vi "ReversedEngineering GetObjectRefsFromPanel.vi"(1 "Path":path, 5 "error in (no error)":errorcluster) -> (15 "objectRefsFound":path[](array[path]), 16 "array":bool[](array[boolean]), 19 "error out":errorcluster)   [LabVIEW 2014]
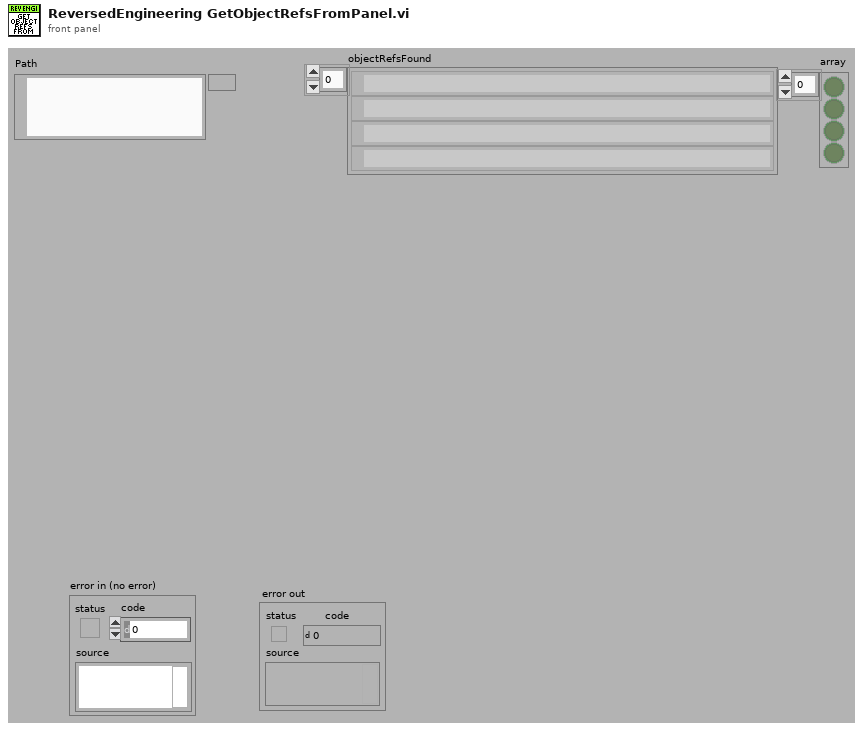
[diagram p1: front panel]
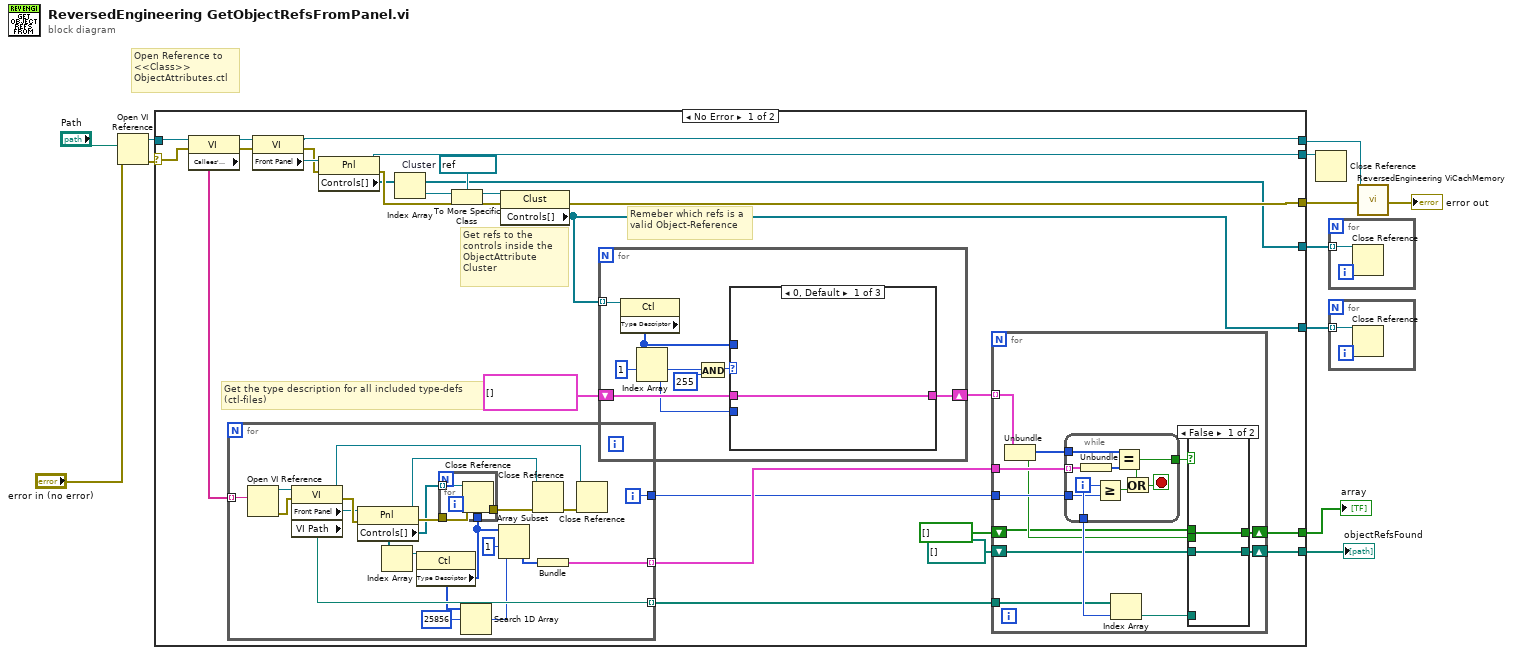
[diagram p0: block diagram]
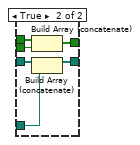
[diagram p2: hidden frame]
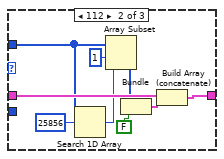
[diagram p3: hidden frame]
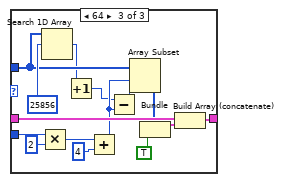
[diagram p4: hidden frame]
diagram:
  # "Open Reference to <<Class>> ObjectAttributes.ctl"
  n1 = Open VI Reference(vi path="Path", error in (no error)="error in (no error)") -> (vi reference=w11:refnum<vi>, error out=w8:errorcluster)  [unwired: 4 out]
  n2 = case shown="No Error" w8 {
    selector: w8 -> [w18 w125]
    tunnel: w11 -> [w37 w124]
    tunnel: [w28 w124] -> w2
    tunnel: [w21 _] -> w9
    tunnel: [w20 w125] -> w3
    tunnel: [w16 _] -> w7
    tunnel: [w15 _] -> w6
    tunnel: [w14 _] -> w5
    tunnel: [w13 _] -> w4
    frame No Error {
      w32 = refnum<vi> refnum  # Cluster
      # "Get the type description for all included type-defs (ctl-files)"
      # "Remeber which refs is a valid Object-Reference"
      # "Get refs to the controls inside the ObjectAttribute Cluster"
      n3 = property class="VI"(reference=w37, error in=w18) -> (reference out=w36:refnum<vi>, error out=w35:errorcluster, "Callees' Names"=w26:string[])
      n4 = for {
        tunnel: w26 -> [w57] mode=indexing
        tunnel: [w51] -> w25 mode=indexing
        tunnel: [w50] -> w23 mode=indexing
        tunnel: [w49] -> w24
        i -> [w49]
        n5 = Open VI Reference(vi path=w57) -> (vi reference=w54:refnum<vi>, error out=w53:errorcluster)  [unwired: 1 in, 4 out]
        n6 = property class="VI"(reference=w54, error in=w53) -> (reference out=w41:refnum<vi>, error out=w56:errorcluster, "Front Panel"=w55:refnum<vi>, "VI Path"=w50:path)
        n7 = property class="Pnl"(reference=w55, error in=w56) -> (reference out=w40:refnum<vi>, error out=w43:errorcluster, "Controls[]"=w39:refnum<vi>[])
        n8 = Index Array(array=w39) -> (element=w52:refnum<vi>)  [unwired: 1 in]
        n9 = property class="Ctl"(reference=w52) -> ("Type Descriptor"=w38:i16[])  [unwired: 1 in, 2 out]
        n10 = for {
          tunnel: [w60] -> w44
          tunnel: w43 -> [w59]
          tunnel: w39 -> [w58] mode=indexing
          tunnel: w38 -> [_]
          n11 = Close Reference(reference=w58, error in (no error)=w59) -> (error out=w60:errorcluster)
        }
        n12 = Search 1D Array(1D array=w38, element=i16 25856) -> (index of element=w45:i32)  [unwired: 1 out]
        n13 = Array Subset(array=w38, index=1, length=w45) -> (w47:i16[])
        n14 = Close Reference(reference=w40, error in (no error)=w44) -> (error out=w42:errorcluster)
        n15 = Bundle(w47) -> (w51:cluster{i16[]})  [unwired: 1 in]
        n16 = Close Reference(reference=w41, error in (no error)=w42) -> ()  [unwired: 1 out]
      }
      n17 = property class="VI"(reference=w36, error in=w35) -> (reference out=w28:refnum<vi>, error out=w29:errorcluster, "Front Panel"=w34:refnum<vi>)
      n18 = property class="Pnl"(reference=w34, error in=w29) -> (reference out=w15:refnum<vi>, error out=w30:errorcluster, "Controls[]"=w14:refnum<vi>[])
      n19 = Index Array(array=w14) -> (element=w33:refnum<vi>)  [unwired: 1 in]
      n20 = To More Specific Class(target class=w32, reference=w33) -> (specific class reference=w31:refnum<vi>)  [unwired: 1 in, 1 out]
      n21 = property class="Clust"(reference=w31, error in=w30) -> (error out=w20:errorcluster, "Controls[]"=w13:refnum<vi>[])  [unwired: 1 out]
      n22 = for {
        tunnel: w13 -> [w98] mode=indexing
        shift-right: [w96] -> w27
        shift-left: cluster{"TypeDesc":i16[], bool}[] [] -> [w97]
        n23 = property class="Ctl"(reference=w98) -> ("Type Descriptor"=w91:i16[])  [unwired: 1 in, 2 out]
        n24 = Index Array(array=w91, index #1=1 ("index")) -> (element #1=w94:i16, element #2=w90:i16)  [unwired: 1 in]
        n25 = And(x=w94, y=i16 255) -> (x .and. y?=w92:i16)
        n26 = case shown="0, Default" w92 {
          tunnel: w97 -> [w99 w108 w123]
          tunnel: [w99 w107 w122] -> w96
          tunnel: w91 -> [_ w101 w114]
          tunnel: w90 -> [_ _ w119]
          frame 0, Default {
          }
          frame 112 {
            n27 = Search 1D Array(1D array=w101, element=i16 25856) -> (index of element=w102:i32)  [unwired: 1 out]
            n28 = Array Subset(array=w101, index=1, length=w102) -> (w105:i16[])
            n29 = Bundle(w105, FALSE) -> (w104:cluster{i16[], bool})  [unwired: 1 out]
            n30 = Build Array (concatenate)(w108, w104) -> (w107:cluster{"TypeDesc":i16[], bool}[])
          }
          frame 64 {
            n31 = Multiply(x=w119, y=i16 2) -> (x*y=w117:i16)
            n32 = Search 1D Array(1D array=w114, element=i16 25856) -> (index of element=w113:i32)  [unwired: 1 out]
            n33 = Increment(x=w113) -> (x+1=w110:i32)
            n34 = Add(x=w117, y=i16 4) -> (x+y=w111:i16)
            n35 = Subtract(x=w110, y=w111) -> (x-y=w112:i32)
            n36 = Array Subset(array=w114, index=w111, length=w112) -> (w121:i16[])
            n37 = Bundle(w121, TRUE) -> (w120:cluster{i16[], bool})  [unwired: 1 out]
            n38 = Build Array (concatenate)(w123, w120) -> (w122:cluster{"TypeDesc":i16[], bool}[])
          }
        }
      }
      n39 = for {
        tunnel: w27 -> [w64] mode=indexing
        tunnel: w25 -> [w73]
        tunnel: w24 -> [w72]
        tunnel: w23 -> [w69]
        shift-right: [w66] -> w21
        shift-left: path[] [] -> [w68]
        shift-right: [w62] -> w16
        shift-left: bool[] [] -> [w61]
        n40 = Unbundle(w64) -> ("TypeDesc"=w65:i16[], w63:bool)
        n41 = while {
          tunnel: w73 -> [w89] mode=indexing
          tunnel: w65 -> [w88]
          tunnel: w72 -> [w85]
          tunnel: [w86] -> w70
          tunnel: [w84] -> w71
          i -> [w86]
          stop <- w82 stop-if-true
          n42 = Unbundle(w89) -> (w87:i16[])
          n43 = Greater Or Equal?(x=w86, y=w85) -> (x >= y?=w83:bool)
          n44 = Equal?(x=w88, y=w87) -> (x = y?=w84:bool)
          n45 = Or(x=w84, y=w83) -> (x .or. y?=w82:bool)
        }
        n46 = Index Array(array=w69, index=w70) -> (element=w67:path)
        n47 = case shown="False" w71 {
          tunnel: [w75 w81] -> w66
          tunnel: w68 -> [w75 w79]
          tunnel: w67 -> [_ w80]
          tunnel: w63 -> [_ w78]
          tunnel: [w74 w77] -> w62
          tunnel: w61 -> [w74 w76]
          frame False {
          }
          frame True {
            n48 = Build Array (concatenate)(w76, w78) -> (w77:bool[])
            n49 = Build Array (concatenate)(w79, w80) -> (w81:path[])
          }
        }
      }
    }
    frame Error {
    }
  }
  "objectRefsFound" <- w9
  "array" <- w7
  n50 = Close Reference(reference=w6) -> ()  [unwired: 1 in, 1 out]
  n51 = for {
    tunnel: w5 -> [w126] mode=indexing
    n52 = Close Reference(reference=w126) -> ()  [unwired: 1 in, 1 out]
  }
  n53 = for {
    tunnel: w4 -> [w127] mode=indexing
    n54 = Close Reference(reference=w127) -> ()  [unwired: 1 in, 1 out]
  }
  n55 = call <resource>:"ReversedEngineering ViCachMemory.vi"("ViRef"=w2, "error in (no error)"=w3) -> ("error out"=→"error out":errorcluster)  [unwired: 2 in, 15 out]
